vi "conversja na string.vi"(5 "max pwm skrecanie":i32, 7 "max obrót":i32, 8 "Z axis":i32, 9 "Y axis":i32, 10 "X axis":i32, 11 "max pwm przod":i32) -> (0 "String 5":string, 1 "String 3":string, 2 "String 2":string, 3 "String 4":string, 4 "String":string)   [LabVIEW 2014]
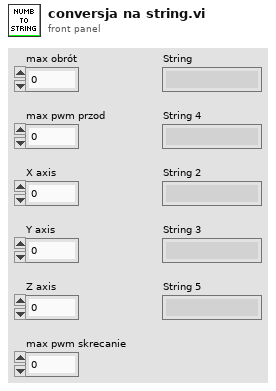
[diagram p1: front panel]
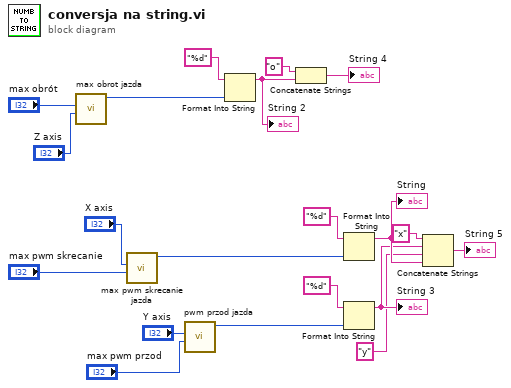
[diagram p0: block diagram]
diagram:
  n1 = call "max obrot jazda.vi"("Z axis"="Z axis", "max obrót"="max obrót") -> ("y"=w13:i32)  [unwired: 9 in]
  n2 = call "max pwm skrecanie jazda.vi"("max pwm skrecanie"="max pwm skrecanie", "X axis"="X axis") -> ("y"=w12:i32)  [unwired: 9 in]
  n3 = call "pwm przod jazda.vi"("max pwm przod"="max pwm przod", "Y axis"="Y axis") -> ("Numeric"=w11:i32)  [unwired: 9 in]
  n4 = Format Into String(format string="%d", w13) -> (resulting string=w9:string)  [unwired: 2 in, 1 out]
  "String 2" <- w9
  n5 = Concatenate Strings("o", w9) -> (→"String 4":string)
  n6 = Format Into String(format string="%d", w12) -> (resulting string=w10:string)  [unwired: 2 in, 1 out]
  "String" <- w10
  n7 = Format Into String(format string="%d", w11) -> (resulting string=w8:string)  [unwired: 2 in, 1 out]
  "String 3" <- w8
  n8 = Concatenate Strings("x", w8, "y", w10) -> (→"String 5":string)
